vi "OpenDevice.vi"(8 "error in (no error)":errorcluster caption="错误输入（无错误）", 9 "nSwitchoverKey":u16, 10 "nAccessMode":u32=1, 11 "handle":u64) -> (0 "error out":errorcluster caption="错误输出", 2 "return":i32, 3 "handle out":u64)   [LabVIEW 2013, in "MvCameraControl.lvlib"]
doc: "MV_LV_API int __stdcall OpenDevice( void* handle,\n unsigned int nAccessMode = 1, \n unsigned short nSwitchoverKey = 0);"
uses:
  MvCameraControl.lvlib
  MvCameraControl.dll
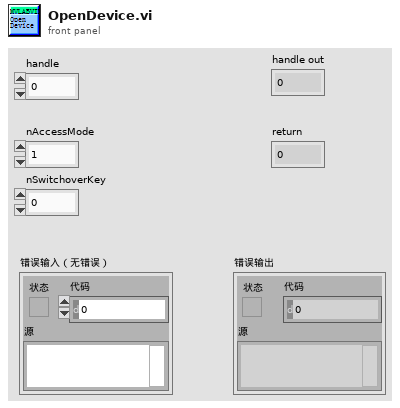
[diagram p1: front panel]
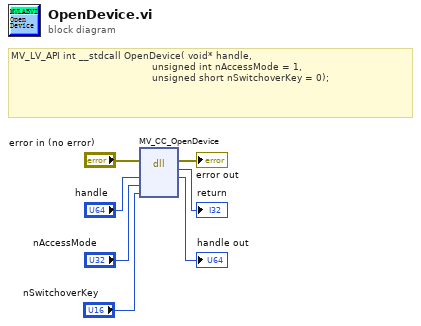
[diagram p0: block diagram]
diagram:
  # "MV_LV_API int __stdcall OpenDevice( void* handle,\n                                               unsigned int nAccessMode = 1, \n                                               unsigned short nSwitchoverKey = 0);"
  n1 = dll-call lib="MvCameraControl.dll" fn="MV_CC_OpenDevice"(error in="error in (no error)", "handle"="handle", "nAccessMode"="nAccessMode", "nSwitchoverKey"="nSwitchoverKey") -> (error out=→"error out":errorcluster, "返回类型"=→"return":i32, "handle"=→"handle out":u64)  [unwired: 4 in, 1 out]
